vi "Create InstrumentStudio Plug-In.vi"() -> ()   [LabVIEW 2021, in "InstrumentStudio Plug-In Editor.lvlib"]
doc: "Tool to generate InstrumentStudio plug-in from template."
uses:
  _InstrumentStudio Plug-In Editor/InstrumentStudio Plug-In Editor.lvlib
  <vilib>/Utility/error.llb/ErrWarn.ctl
  _InstrumentStudio Plug-In Editor/Data Holder.ctl
panel:
  in  "Group":string caption="InstrumentStudio Plug-in Group"
  out "Status":T1=TRUE caption="InstrumentStudio plug-in name must be unique and cannot contain any of the following characters:\n           \\ / : * ? \" < > |"
  in  "Create InstrumentStudio Plug-in":bool
  in  "Name":string caption="InstrumentStudio Plug-in Name"
  out "Active Project Name":string
  # "* Project in which the InstrumentStudio plug-in will be created"
  # "* Group under which the plug-in will be populated in the Add-Ons\ncategory of InstrumentStudio's Edit Layout Dialog"
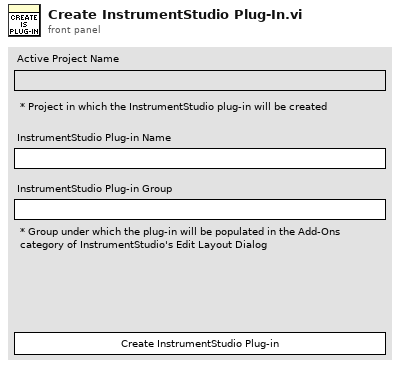
[diagram p1: front panel]
types:
  T1 = typedef "ErrWarn.ctl" = bool
  T2 = enum8{"Enabled", "Disabled", "Disabled and Grayed Out"}
  T3 = typedef "InstrumentStudio Plug-In Editor.lvlib/Data Holder.ctl" = cluster{"project refnum":refnum<vi>, "plugin name":string, "plugin group name":string}
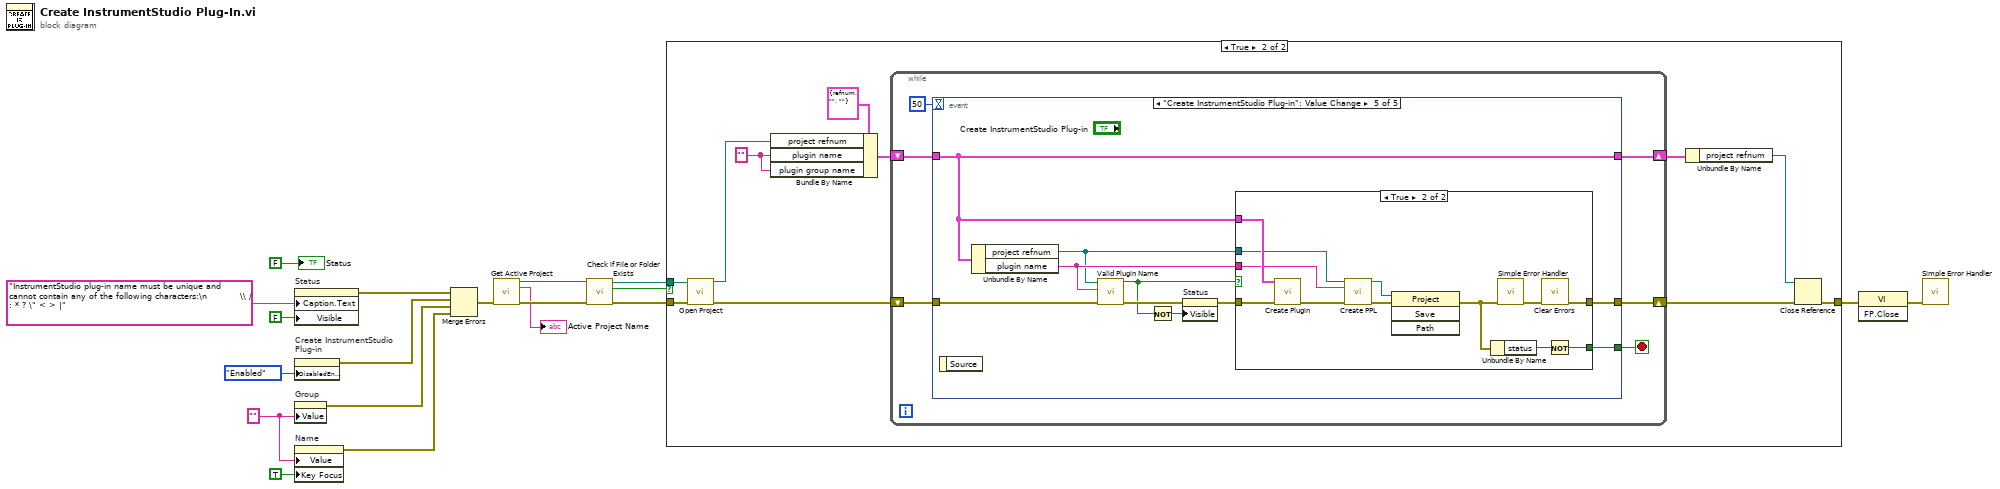
[diagram p0: block diagram]
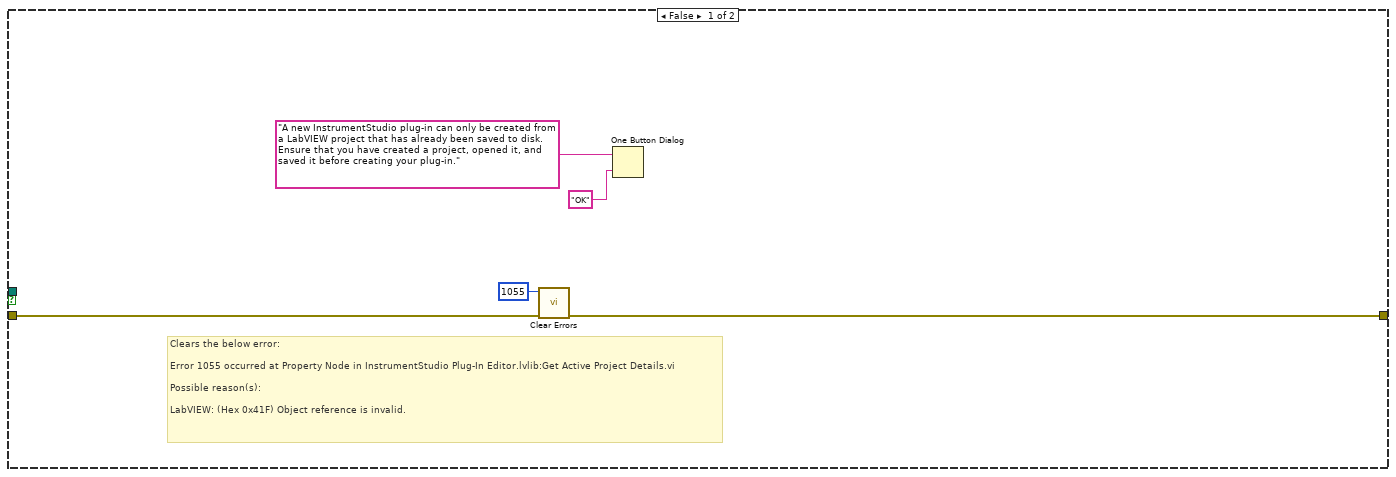
[diagram p2: hidden frame]
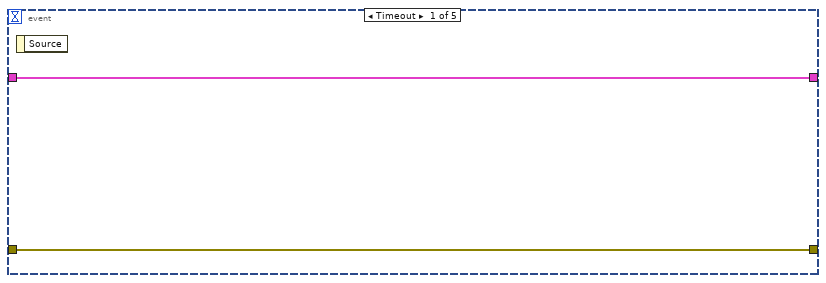
[diagram p3: hidden frame]
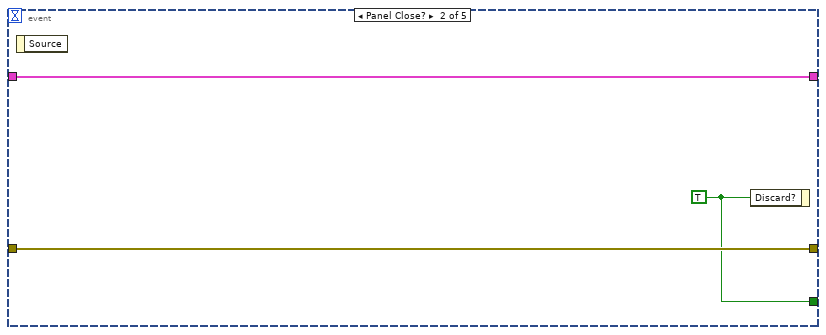
[diagram p4: hidden frame]
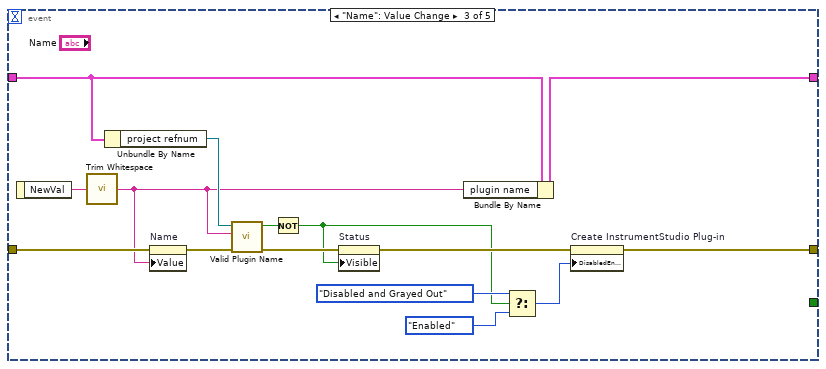
[diagram p5: hidden frame]
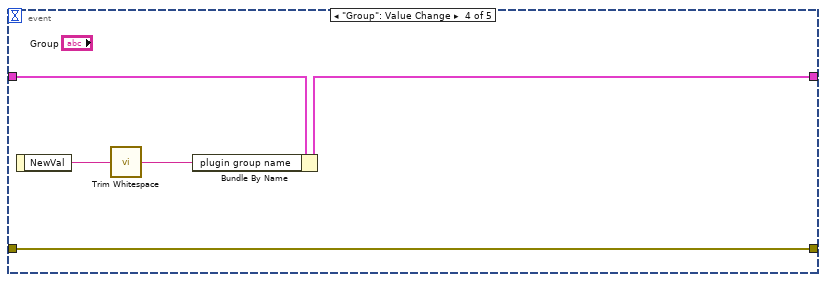
[diagram p6: hidden frame]
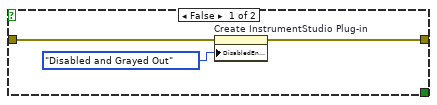
[diagram p7: hidden frame]
diagram:
  w5 = "" ("Group")
  n1 = property on="Status" class="Bool"("Caption.Text"="InstrumentStudio plug-in name must be unique and cannot contain any of the following characters:\n           \\ / : * ? \" < > |" ("Status"), "Visible"=FALSE) -> (error out=w11:errorcluster)  [unwired: 2 in, 1 out]
  n2 = property on="Create InstrumentStudio\nPlug-in" class="Bool"("DisabledEnum"=T2."Enabled" ("Disabled")) -> (error out=w10:errorcluster)  [unwired: 2 in, 1 out]
  n3 = property on="Group" class="Str"("Value"=w5) -> (error out=w9:errorcluster)  [unwired: 2 in, 1 out]
  n4 = property on="Name" class="Str"("Value"=w5, "Key Focus"=TRUE) -> (error out=w8:errorcluster)  [unwired: 2 in, 1 out]
  n5 = Merge Errors(w11, w10, w9, w8) -> (w7:errorcluster)
  n6 = call "Get Active Project.vi"("error in"=w7) -> ("path"=w14:path, "name"=→"Active Project Name":string, "error out"=w15:errorcluster)  [unwired: 12 in]
  n7 = call <vilib>:"Check if File or Folder Exists.vi"("error in (no error)"=w15, "path"=w14) -> ("error out"=w17:errorcluster, "file or folder exists?"=w12:bool, "dup path"=w16:path)  [unwired: 7 in]
  n8 = case shown="True" w12 {
    tunnel: w17 -> [w22 w34]
    tunnel: [w21 w27] -> w18
    tunnel: w16 -> [_ w26]
    frame False {
      # "Clears the below error:\n\nError 1055 occurred at Property Node in InstrumentStudio Plug-In Editor.lvlib:Get Active Project Details.vi\n\nPossible reason(s):\n\nLabVIEW: (Hex 0x41F) Object reference is invalid."
      n9 = call <vilib>:"Clear Errors.vi"("error in (no error)"=w22, "specific error code to clear (0: all)"=1055) -> ("error out"=w21:errorcluster)  [unwired: 4 in, 1 out]
      n10 = One Button Dialog(message="A new InstrumentStudio plug-in can only be created from a LabVIEW project that has already been saved to disk.  Ensure that you have created a project, opened it, and saved it before creating your plug-in.", button name ("OK")="OK") -> ()  [unwired: 1 out]
    }
    frame True {
      w25 = ""
      n11 = call "Open Project.vi"("project path"=w26, "error in"=w34) -> ("project refnum"=w32:refnum<vi>, "error out"=w35:errorcluster)  [unwired: 12 in]
      n12 = Bundle By Name(cluster=T3 {"project refnum"=refnum, "plugin name"="", "plugin group name"=""}, "project refnum"=w32, "plugin name"=w25, "plugin group name"=w25) -> (w31:T3)
      n13 = while {
        shift-right: [w38] -> w28
        shift-left: w35 -> [w41]
        shift-right: [w39] -> w30
        shift-left: w31 -> [w40]
        stop <- w36 stop-if-true
        n14 = event shown="[4] \"Create InstrumentStudio Plug-in\": Value Change" {
          selector: _ -> [_ _ _ _ _]
          dyn-events: _ -> [_ _ _ _ _]
          timeout: 50 -> [_ _ _ _ _]
          tunnel: w41 -> [w42 w45 w55 w65 w76]
          tunnel: w40 -> [w43 w46 w59 w66 w71]
          tunnel: [w43 w46 w60 w64 w71] -> w39
          tunnel: [w42 w45 w52 w65 w73] -> w38
          tunnel: [_ w44 _ _ w69] -> w36
          event Timeout {
            n15 = event-data() -> ()  [unwired: 1 in, 1 out]
          }
          event Panel Close? {
            w44 = TRUE ("Discard?")
            n16 = event-data() -> ()  [unwired: 1 in, 1 out]
            n17 = event-data("Discard?"=w44) -> ()  [unwired: 1 in, 1 out]
          }
          event "Name": Value Change {
            n18 = event-data() -> ("NewVal"=w61:string)  [unwired: 1 in]
            n19 = call <vilib>:"Trim Whitespace.vi"("string"=w61) -> ("trimmed string"=w54:string)  [unwired: 1 in]
            n20 = Unbundle By Name(w59) -> ("project refnum"=w58:refnum<vi>)
            n21 = property on="Name" class="Str"(error in=w55, "Value"=w54) -> (error out=w56:errorcluster)  [unwired: 1 in, 1 out]
            n22 = call "Valid Plugin Name.vi"("error in"=w56, "requested plugin name"=w54, "project refnum"=w58) -> ("error out"=w57:errorcluster, "valid name?"=w53:bool)  [unwired: 7 in]
            n23 = Not(x=w53) -> (.not. x?=w47:bool)
            n24 = property on="Status" class="Bool"(error in=w57, "Visible"=w47) -> (error out=w51:errorcluster)  [unwired: 1 in, 1 out]
            n25 = Bundle By Name(cluster=w59, "plugin name"=w54) -> (w60:T3)
            n26 = Select(t=T2."Disabled and Grayed Out" ("Disabled"), s=w47, f=T2."Enabled" ("Disabled")) -> (s? t:f=w48:T2)
            n27 = property on="Create InstrumentStudio Plug-in" class="Bool"(error in=w51, "DisabledEnum"=w48) -> (error out=w52:errorcluster)  [unwired: 1 in, 1 out]
          }
          event "Group": Value Change {
            n28 = event-data() -> ("NewVal"=w63:string)  [unwired: 1 in]
            n29 = call <vilib>:"Trim Whitespace.vi"("string"=w63) -> ("trimmed string"=w62:string)  [unwired: 1 in]
            n30 = Bundle By Name(cluster=w66, "plugin group name"=w62) -> (w64:T3)
          }
          event "Create InstrumentStudio Plug-in": Value Change {
            n31 = event-data() -> ()  [unwired: 1 in, 1 out]
            n32 = Unbundle By Name(w71) -> ("project refnum"=w67:refnum<vi>, "plugin name"=w72:string)
            n33 = call "Valid Plugin Name.vi"("error in"=w76, "requested plugin name"=w72, "project refnum"=w67) -> ("error out"=w75:errorcluster, "valid name?"=w68:bool)  [unwired: 7 in]
            n34 = Not(x=w68) -> (.not. x?=w70:bool)
            n35 = property on="Status" class="Bool"(error in=w75, "Visible"=w70) -> (error out=w74:errorcluster)  [unwired: 1 in, 1 out]
            n36 = case shown="True" w68 {
              tunnel: w74 -> [w79 w91]
              tunnel: [w78 w86] -> w73
              tunnel: w72 -> [_ w83]
              tunnel: [_ w84] -> w69
              tunnel: w71 -> [_ w88]
              tunnel: w67 -> [_ w80]
              frame False {
                n37 = property on="Create InstrumentStudio Plug-in" class="Bool"(error in=w79, "DisabledEnum"=T2."Disabled and Grayed Out" ("Disabled")) -> (error out=w78:errorcluster)  [unwired: 1 in, 1 out]
              }
              frame True {
                n38 = call "Create Plugin.vi"("configuration"=w88, "error in"=w91) -> ("error out"=w90:errorcluster)  [unwired: 13 in]
                n39 = call "Create PPL.vi"("project refnum in"=w80, "plug-in name"=w83, "error in (no error)"=w90) -> ("project refnum out"=w82:refnum<vi>, "error out"=w89:errorcluster)  [unwired: 11 in]
                n40 = invoke class="Project" method="Save"(reference=w82, error in=w89) -> (error out=w81:errorcluster)  [unwired: 2 in, 3 out]
                n41 = Unbundle By Name(w81) -> ("status"=w85:bool)
                n42 = call <vilib>:"Simple Error Handler.vi"("error in (no error)"=w81) -> ("error out"=w87:errorcluster)  [unwired: 4 in, 4 out]
                n43 = call <vilib>:"Clear Errors.vi"("error in (no error)"=w87) -> ("error out"=w86:errorcluster)  [unwired: 5 in, 1 out]
                n44 = Not(x=w85) -> (.not. x?=w84:bool)
              }
            }
          }
        }
      }
      n45 = Unbundle By Name(w30) -> ("project refnum"=w29:refnum<vi>)
      n46 = Close Reference(reference=w29, error in (no error)=w28) -> (error out=w27:errorcluster)
    }
  }
  n47 = invoke class="VI" method="FP.Close"(error in=w18) -> (error out=w19:errorcluster)  [unwired: 2 in, 2 out]
  n48 = call <vilib>:"Simple Error Handler.vi"("error in (no error)"=w19) -> ()  [unwired: 4 in, 5 out]
  "Status" <- T1 FALSE ("Status")
